vi "GlobalFrameCntr.vi"() -> ()   [LabVIEW 2010]
panel:
  in  "frame cntr":u32
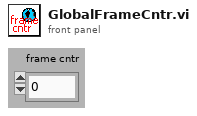
[diagram p1: front panel]
diagram:
